vi "Create Client.vi"(8 "error in":errorcluster, 11 "cluster id":string) -> (0 "error out":errorcluster, 3 "grpc client id":T1)   [LabVIEW 2020, in "MeasurementLink Discovery V1.lvlib"]
uses:
  MeasurementLink Discovery V1.lvlib
  <vilib>/gRPC/LabVIEW gRPC Library/Shared/grpcId.ctl
  Generated/Measurement Plugin Discovery Client/Measurement Plugin Discovery Client.lvlib
  <vilib>/gRPC/LabVIEW gRPC Library/grpc-lvsupport-release.lvlib
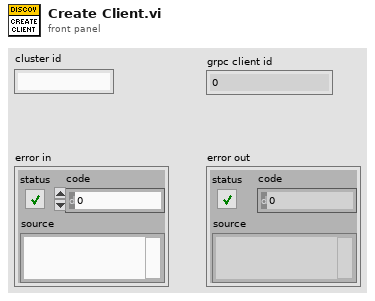
[diagram p1: front panel]
types:
  T1 = typedef "grpc-lvsupport-release.lvlib/grpcId.ctl" = u64
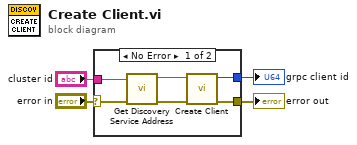
[diagram p0: block diagram]
diagram:
  n1 = case shown="No Error" "error in" {
    selector: "error in" -> [w8 w11]
    tunnel: [w10 _] -> w4
    tunnel: [w9 w11] -> w3
    tunnel: "cluster id" -> [w5 _]
    frame No Error {
      n2 = call "Get Discovery Service Address.vi"("error in"=w8, "cluster id (\"\")"=w5) -> ("error out"=w6:errorcluster, "address"=w7:string)  [unwired: 8 in]
      n3 = call "Create Client.vi"("error in"=w6, "address"=w7) -> ("error out"=w9:errorcluster, "gRPC ID Out"=w10:T1)  [unwired: 8 in]
    }
    frame Error {
    }
  }
  "grpc client id" <- w4
  "error out" <- w3
